vi "Reset flashing button.vi"(8 "error in (no error)":errorcluster, 9 "Digital Values":T1[](array[typedef]), 10 "Digital Signal Index":i32, 11 "Controll collection":T2) -> (0 "error out":errorcluster)   [LabVIEW 2011]
uses:
  Controll refrence groups.ctl
  Measurments Handling/Status Digitalish.ctl
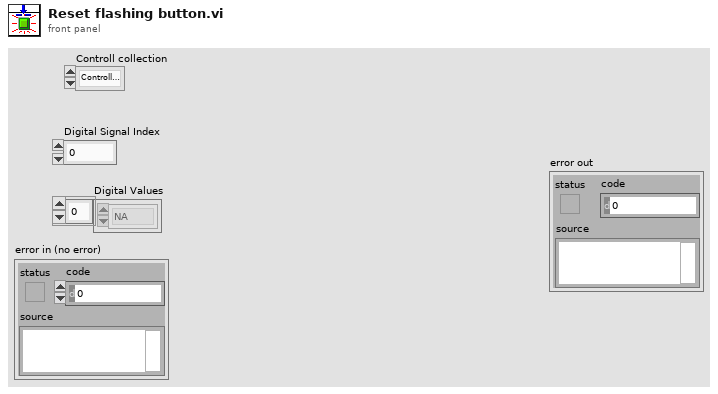
[diagram p1: front panel]
types:
  T1 = typedef "Status Digitalish.ctl" = enum16{"NA", "False", "True"}
  T2 = typedef "Controll refrence groups.ctl" = enum16{"Controller. gen", "Controller . High G", "Stroker", "PCP Online", "PCP Local", "PCP HV On", "Driller", "Stroker Cmd Buttons", "Stroker Anchor Cmd Buttons", "Controller Relay Buttons", "PCP Start Telemetry", "PCP Start Motor", "Tractor", "Modem Status"}
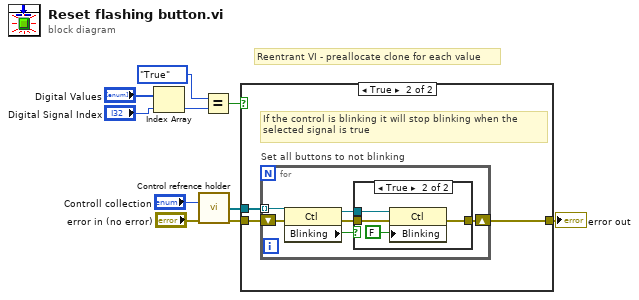
[diagram p0: block diagram]
diagram:
  # "Reentrant VI - preallocate clone for each value"
  n1 = Index Array(array="Digital Values", index="Digital Signal Index") -> (element=w2:T1)
  n2 = call "Control refrence holder.vi"("Controll collection"="Controll collection", "error in (no error)"="error in (no error)") -> ("Controlls out"=w9:refnum<vi>[], "error out"=w8:errorcluster)  [unwired: 12 in]
  n3 = Equal?(x=Status_Digitalish."True", y=w2) -> (x = y?=w1:bool)
  n4 = case shown="True" w1 {
    tunnel: w9 -> [_ w14]
    tunnel: w8 -> [w11 w13]
    tunnel: [w11 w12] -> w6
    frame False {
    }
    frame True {
      # "If the control is blinking it will stop blinking when the \nselected signal is true"
      n5 = for "Set all buttons to not blinking" {
        tunnel: w14 -> [w20] mode=indexing
        shift-right: [w15] -> w12
        shift-left: w13 -> [w19]
        n6 = property on="Property Node" class="Ctl"(reference=w20, error in=w19) -> (reference out=w16:refnum<vi>, error out=w17:errorcluster, "Blinking"=w18:bool)
        n7 = case shown="True" w18 {
          tunnel: w17 -> [w21 w23]
          tunnel: w16 -> [_ w24]
          tunnel: [w21 w22] -> w15
          frame False {
          }
          frame True {
            n8 = property on="Property Node" class="Ctl"(reference=w24, error in=w23, "Blinking"=FALSE) -> (error out=w22:errorcluster)  [unwired: 1 out]
          }
        }
      }
    }
  }
  "error out" <- w6
